vi "read_data.vi"(8 "error in (no error)":errorcluster, 10 "bytes to read":i32, 11 "DL090602SutterMP285Stage in":refnum<class "StageDL090602SutterMP285.lvclass">) -> (0 "error out":errorcluster, 2 "hex data string":string, 3 "DL090602SutterMP285Stage out":refnum<class "StageDL090602SutterMP285.lvclass">)   [LabVIEW 2010, in "StageDL090602SutterMP285.lvclass"]
uses:
  StageDL090602SutterMP285.lvclass
  StageDL090602SutterMP285.lvclass/StageDL090602SutterMP285.ctl
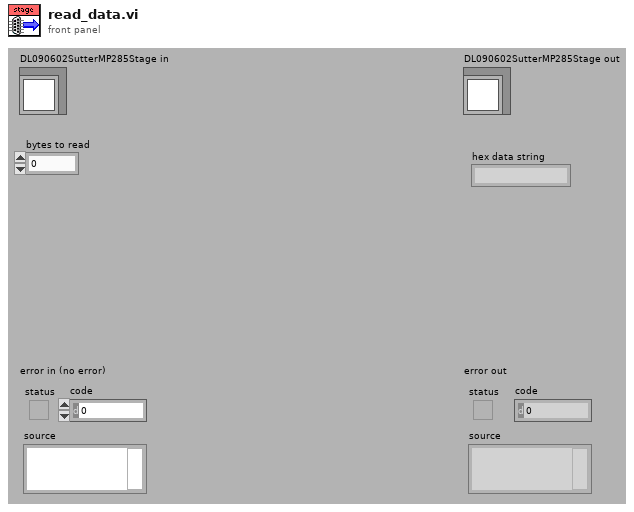
[diagram p1: front panel]
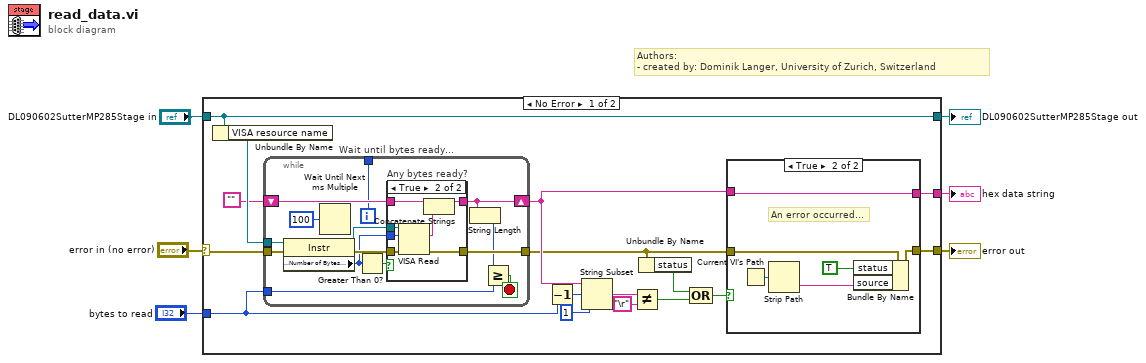
[diagram p0: block diagram]
diagram:
  # "Authors: \n- created by: Dominik Langer, University of Zurich, Switzerland"
  n1 = case shown="No Error" "error in (no error)" {
    selector: "error in (no error)" -> [w12 w55]
    tunnel: [w18 w55] -> w6
    tunnel: [w7 w54] -> w4
    tunnel: "DL090602SutterMP285Stage in" -> [w7 w54]
    tunnel: [w17 _] -> w3
    tunnel: "bytes to read" -> [w8 _]
    frame No Error {
      n2 = Unbundle By Name(w7) -> ("VISA resource name"=w13:refnum<visa-resource-name>)
      n3 = while "Wait until bytes ready..." {
        tunnel: w13 -> [w36]
        tunnel: w12 -> [w35]
        tunnel: [w31] -> w10
        tunnel: w8 -> [w27]
        shift-right: [w29] -> w11
        shift-left: "" -> [w30]
        tunnel: [w23] -> _
        i -> [w23]
        stop <- w26 stop-if-true
        n4 = property class="Instr"(reference=w36, error in=w35) -> (reference out=w32:refnum<visa-resource-name>, error out=w33:errorcluster, "Serial Settings:Number of Bytes at Serial Port"=w24:u32)
        n5 = Wait Until Next ms Multiple(millisecond multiple=u32 100) -> ()  [unwired: 1 out]
        n6 = Greater Than 0?(x=w24) -> (x > 0?=w25:bool)
        n7 = case "Any bytes ready?" shown="True" w25 {
          tunnel: w33 -> [w38 w45]
          tunnel: w32 -> [_ w44]
          tunnel: [w38 w43] -> w31
          tunnel: w30 -> [w37 w42]
          tunnel: [w37 w40] -> w29
          tunnel: w24 -> [_ w39]
          frame False {
          }
          frame True {
            n8 = VISA Read(VISA resource name=w44, byte count=w39, error in (no error)=w45) -> (read buffer=w41:string, error out=w43:errorcluster)  [unwired: 2 out]
            n9 = Concatenate Strings(w42, w41) -> (w40:string)
          }
        }
        n10 = String Length(string=w29) -> (length=w28:i32)
        n11 = Greater Or Equal?(x=w28, y=w27) -> (x >= y?=w26:bool)
      }
      n12 = Decrement(x=w8) -> (x-1=w22:i32)
      n13 = String Subset(string=w11, offset (0)=w22, length (rest)=1 ("length (rest)")) -> (substring=w20:string)
      n14 = Not Equal?(x=w20, y="\r") -> (x != y?=w16:bool)
      n15 = Unbundle By Name(w10) -> ("status"=w15:bool)
      n16 = Compound Arithmetic op=OR(w15, w16) -> (w14:bool)
      n17 = case shown="True" w14 {
        tunnel: w10 -> [w47 w53]
        tunnel: [w47 w52] -> w18
        tunnel: [w46 w48] -> w17
        tunnel: w11 -> [w46 w48]
        frame False {
          # "No error..."
        }
        frame True {
          # "An error occurred..."
          n18 = Current VI's Path() -> (path=w50:path)
          n19 = Strip Path(path=w50) -> (name=w49:string)  [unwired: 1 out]
          n20 = Bundle By Name(cluster=w53, "status"=TRUE, "source"=w49) -> (w52:errorcluster)
        }
      }
    }
    frame Error {
    }
  }
  "error out" <- w6
  "DL090602SutterMP285Stage out" <- w4
  "hex data string" <- w3
